vi "Dashboard Main.vi"() -> ()   [LabVIEW 2018]
uses:
  <vilib>/Utility/miscctls.llb/LVRowAndColumnTypeDef.ctl
  <vilib>/event_ctls.llb/eventvkey.ctl
  <vilib>/Rock Robotics/Network Tables/NT Read Numeric Array.vi
  <vilib>/Rock Robotics/WPI/Dashboard/WPI_DashboardLogging Global.vi
panel:
  in  "Camera Settings Right":T1={"Frame Rate"=30, "Compression"=30, "Size"=1, "DB Camera Config"=FALSE} {"Frame Rate" scale=1.0..30.0; "Compression" scale=100.0..-1.0; "Size" items=["640x480", "320x240", "160x120"]}
  in  "Camera Name Right":string(combo)="No Camera Selection"
  out "Camera Perf":string
  in  "Camera Settings":T1={"Frame Rate"=30, "Compression"=30, "Size"=1, "DB Camera Config"=FALSE} {"Frame Rate" scale=1.0..30.0; "Compression" scale=100.0..-1.0; "Size" items=["640x480", "320x240", "160x120"]}
  in  "TCP":refnum<k5>
  in  "Rec Mode":enum32{"Stop", "Record", "Playback"}(radio)
  out "Robot IP":string
  out "Image Message":string="Timeout in Camera Communications"
  in  "Dashboard Tab":T2(tab)
  in  ".Avg Factor":i32=20
  in  "Recognition Limits":T3={"x1 (L) low"=31.0, "x1 (L) high"=71.0, "y1 (L) low "=131.0, "y1 (L) high"=171.0, "x2 (L) low"=249.0, "x2 (L) high"=289.0, "y2 (L) low"=133.0, "y2 (L) high"=173.0}
  out "y1 (L)":dbl
  out "x1 (L)":dbl
  in  "Enable Vision\nProcessing":bool
  out "y2 (R)":dbl
  out "x2 (L)":dbl
  in  "Photo\nStore Rate":u32=100
  in  "Reset":bool
  in  "# New Images\nto Store":i32=1
  in  "Start\nStoring":bool
  out "Total Stored\nSince Reset":i32
  in  "Select Auto":string(combo)="Select Autonomous ..."
  out "NT Connection":bool
  out "MotorChart R":cluster{"Numeric":dbl, "Numeric":dbl}(graph)
  out "MotorChart L":cluster{"Numeric":dbl, "Numeric":dbl}(graph)
  out "MotorSliders R":cluster{"MotorSlide1":dbl, "MotorSlide2":dbl} {"MotorSlide2" scale=-1.0..1.0 scale format="%#_2e"; "MotorSlide1" scale=-1.0..1.0 scale format="%#_2e"}
  out "MotorSliders L":cluster{"MotorSlide1":dbl, "MotorSlide2":dbl} {"MotorSlide2" scale=-1.0..1.0 scale format="%#_2e"; "MotorSlide1" scale=-1.0..1.0 scale format="%#_2e"}
  out "Gyro":dbl(knob) scale=0.0..360.0
  out "JS1 Z":dbl(slide) scale=-1.0..1.0 scale format="%#_2e"
  out "JS1 Graph":cluster{"X":dbl, "Y":dbl}[](graph)
  out "JS1 Buttons":T4
  out "JS2 Z":dbl(slide) scale=-1.0..1.0 scale format="%#_2e"
  out "JS2 Graph":cluster{"X":dbl, "Y":dbl}[](graph)
  out "JS2 Buttons":T4
  out "Mode":T5(ring)=enum."Auto Disabled"
  out "Right Camera Perf":cluster{"Bandwidth (Mbps)":dbl, "FPS":dbl}
  out "Camera Image Right":T6(plugin-control)
  in  "DB/String 9":string
  in  "DB/String 8":string
  in  "DB/String 7":string
  in  "DB/String 6":string
  in  "DB/String 5":string
  in  "DB/String 4":string
  in  "DB/String 3":string
  in  "DB/String 2":string
  in  "DB/String 1":string
  in  "DB/String 0":string
  in  "DB/Slider 0":dbl(slide) scale=0.0..5.0
  in  "DB/Slider 1":dbl(slide) scale=0.0..5.0
  in  "DB/Slider 2":dbl(slide) scale=0.0..5.0
  in  "DB/Slider 3":dbl(slide) scale=0.0..5.0
  out "DB/LED 3":bool
  out "DB/LED 2":bool
  out "DB/LED 1":bool
  out "DB/LED 0":bool
  in  "DB/Button 3":bool
  in  "DB/Button 2":bool
  in  "DB/Button 1":bool
  in  "DB/Button 0":bool caption="New Name"
  in  "Test Slider":dbl(slide) scale=0.0..100.0 scale format="%#_3g"
  in  "On/Off":bool caption="Solenoid"
  in  "Test Name":u16(ring) items=["Select the test to run..."]
  in  "Test Tree":string(tree)
  in  "Motor":cluster{"Value":dbl, "Enable":bool} {"Value" scale=-1.0..1.0 scale format="%#_3g"}
  out "Progress":T7 {"Test Progress" scale=0.0..100.0}
  in  "Rev/Fwd":cluster{"Forward":bool, "Reverse":bool}
  in  "Test Ring":u16(ring) items=["Monochrome", "Color"]
  out "Cmd Status":string
  in  "Execute Command":bool
  in  "Command Params":string[][](table)
  in  "Command Selection":i32(listbox)
  in  "CheckList":i32(listbox)
  out "Tree":string(tree)
  out "Camera Image":T6(plugin-control)
  out "Background":bool
  in  "Camera Name":string(combo)="No Camera Selection"
  # "HW"
  # "HW"
  # "Joysticks"
  # "Drive Motors"
  # "Front"
  # "Right"
  # "Left"
  # "Back"
  # "This tab is a great place for autonomous settings and robot-specific values.\nPlace controls and indicators inside this tab and match name to\nDashboard Variables on robot. You can also delete this comment."
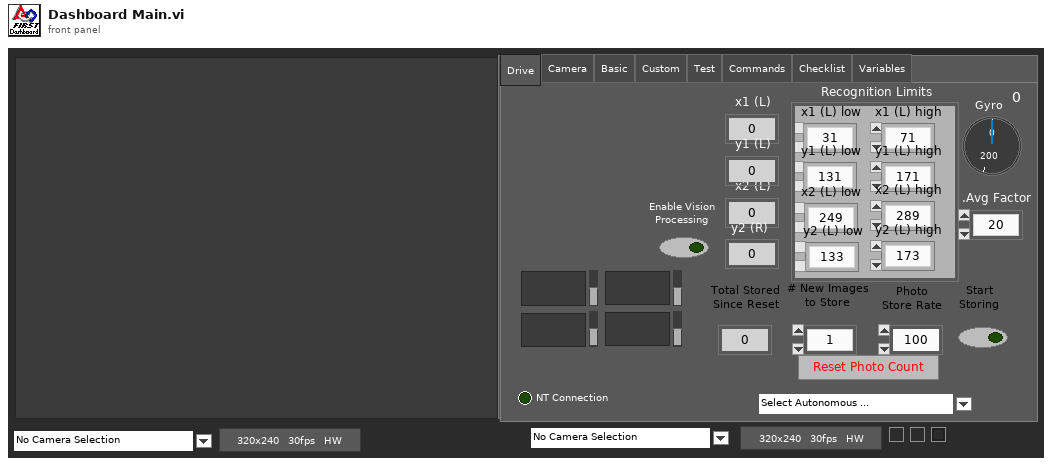
[diagram p1: front panel]
types:
  T1 = cluster{"Frame Rate":i32, "Compression":i32, "Size":u16, "DB Camera Config":bool}
  T2 = enum32{"Drive", "Camera", "Basic", "Custom", "Test", "Commands", "Checklist", "Variables"}
  T3 = cluster{"x1 (L) low":dbl, "x1 (L) high":dbl, "y1 (L) low ":dbl, "y1 (L) high":dbl, "x2 (L) low":dbl, "x2 (L) high":dbl, "y2 (L) low":dbl, "y2 (L) high":dbl}
  T4 = cluster{bool, bool, bool, bool, bool, bool, bool, bool, bool, bool, bool, bool}
  T5 = enum8{"Tele-Op Disabled", "Tele-Op Enabled", "Auto Disabled", "Auto Enabled", "Test Disabled", "Test Enabled", "Disconnected", "No Code", "E-Stop"}
  T6 = typedef "IMAQ Image.ctl" = refnum<image>
  T7 = cluster{"Test Progress":u8, "Test Progress Text":string}
  T8 = cluster{"Save Path":path, "Interval (s)":dbl, "Keep":i32}
  T9 = typedef "Image Type" = u32
  T10 = cluster{"IDs":cluster{"RPC field ID":u16, "Unique ID":u16}, "String":string}
  T11 = cluster{"Error Strings":string, "Disable Counts":cluster{u16, u16}, "Rail Faults":cluster{u16, u16, u16}, "Robot IP":string, "DB Mode":u8, "Event Info":cluster{"Name":string, "Type":u8, "Number":u16, "Replay":u8}}
  T12 = cluster{"Storage":cluster{"Disk Free":u64, "RAM Block":u32, "RAM free":u32}, "CPU Utilization":cluster{"CPU % ISR":sgl, "CPU % Time Crit":sgl, "CPU % Timed Str":sgl, "CPU % High":sgl, "CPU % Above":sgl, "CPU % Normal":sgl, "CPU % Low":sgl}, "CAN":cluster{"% Bus Utilization":sgl, "Bus Off Cnt":u32, "TX_FIFO Full Cnt":u32, "Receive Error Cnt":u8, "Transmit Error Cnt":u8}, "HID":cluster{"HID Outputs":u32, "Rumble Low":u16, "Rumble High":u16}[]}
  T13 = cluster{"Status bits":cluster{"Test Mode":bool, "Autonomous":bool, "Enabled":bool, "Code Start":bool, "Brownout":bool, "Reserved 2":bool, "Reserved 3":bool, "E-Stop":bool}, "Code Trace":cluster{"Disabled":bool, "TeleOp":bool, "Auto":bool, "Test":bool}, "Controller Type":enum16{"unknown", "cRIO", "roboRio"}, "Code?":enum16{"unknown", "noCode", "code"}, "Battery V":dbl}
  T14 = cluster{"Control Bits":cluster{"TestMode":bool, "Autonomous":bool, "Enabled":bool, "FMS Present":bool, bool, bool, bool, "E-Stop":bool}, "Team Station ":u8, "Countdown":sgl, "Joystick Values":cluster{"Axes":dbl[], "Buttons":bool[], "POVs":i16[]}[]}
  T15 = cluster{"Axes":dbl[], "Buttons":bool[], "POVs":i16[]}[]
  T16 = cluster{"Axes":dbl[], "Buttons":bool[], "POVs":i16[]}
  T17 = cluster{"Buttons[0]":bool, "Buttons[1]":bool, "Buttons[2]":bool, "Buttons[3]":bool, "Buttons[4]":bool, "Buttons[5]":bool, "Buttons[6]":bool, "Buttons[7]":bool, "Buttons[8]":bool, "Buttons[9]":bool, "Buttons[10]":bool, "Buttons[11]":bool}
  T18 = cluster{"Camera Image":refnum<vi>, "Dashboard Tab":refnum<vi>, "Background":refnum<vi>, "Rec Mode":refnum<vi>, "Test Slider":refnum<vi>, "On/Off ":refnum<vi>, "Test Ring":refnum<vi>, "Rev/Fwd":refnum<vi>, "Test Name":refnum<vi>, "Motor":refnum<vi>, "Progress":refnum<vi>, "CheckList":refnum<vi>, "Tree":refnum<vi>, "Test Tree":refnum<vi>, "Command Params":refnum<vi>, "Command Selection":refnum<vi>, "Execute Command":refnum<vi>, "Cmd Status":refnum<vi>, "Camera Settings":refnum<vi>, "Camera Name":refnum<vi>, "Camera Perf":refnum<vi>, "Camera Settings Right":refnum<vi>, "Camera Name Right":refnum<vi>, "Camera Image Right":refnum<vi>}
  T19 = cluster{"Global Rectangle":i32[], "Contours":cluster{"Contour Type":u32, "ROI Type":u32, "Points":i32[]}[]}
  T20 = cluster{"Camera Name":string, string, "Saved DB Images Info":cluster{"Save Path":path, "Interval (s)":dbl, "Keep":i32}}
  T21 = cluster{"Position":cluster{"x":sgl, "y":sgl}, "Angle":sgl, "Scale":sgl, "Score":sgl, "Bounding Box":cluster{"x":sgl, "y":sgl}[]}[]
  T22 = typedef "IMAQ GM Match Report.ctl" = cluster{"Position":cluster{"x":sgl, "y":sgl}, "Angle":sgl, "Scale":sgl, "Score":sgl, "Bounding Box":cluster{"x":sgl, "y":sgl}[], "Contrast Reversed":bool, "Occlusion %":sgl, "Template Target Curve Score":sgl, "Target Template Curve Score":sgl, "Correlation Score":sgl}
  T23 = cluster{"Position":cluster{"x":sgl, "y":sgl}, "Angle":sgl, "Scale":sgl, "Score":sgl, "Bounding Box":cluster{"x":sgl, "y":sgl}[]}
  T24 = cluster{"Camera Name Right":string, string, "Saved DB Images Info":cluster{"Save Path":path, "Interval (s)":dbl, "Keep":i32}}
  T25 = cluster{"Operation":enum16{"Update", "Clear"}, "Color Box":u32}[]
  T26 = typedef "eventvkey.ctl" = enum16{"ASCII", "Enter", "Return", "Shift", "Ctrl", "Alt", "Cmd", "Opt", "Caps", "NumLock", "Clear", "Break", "Up", "Down", "Left", "Right", "Insert", "Delete", "Home", "End", "PageUp", "PageDown", "Escape", "Help", "Pause", "ScrollLock", "F1", "F2", "F3", "F4", "F5", "F6", "F7", "F8", "F9", "F10", "F11", "F12", "F13", "F14", "F15", "F16", "F17", "F18", "F19", "F20", "F21", "F22", "F23", "F24", "Play", "VolumeUp", "VolumeDown", "Mute", "Two Byte Char"}
  T27 = cluster{"Image Size":bool, "Image Type":bool, "Pixel Value":bool, "ROI Information":bool, "Zoom Factor":bool}
  T28 = cluster{"Operation":enum16{"Update", "Clear"}, "Color Box":u32}
  T29 = typedef "LVRowAndColumnTypeDef.ctl" = cluster{"Row":i32, "Column":i32}
  T30 = cluster{"Shift":bool, "Ctrl":bool, "Alt":bool, "Cmd":bool, "Opt":bool}
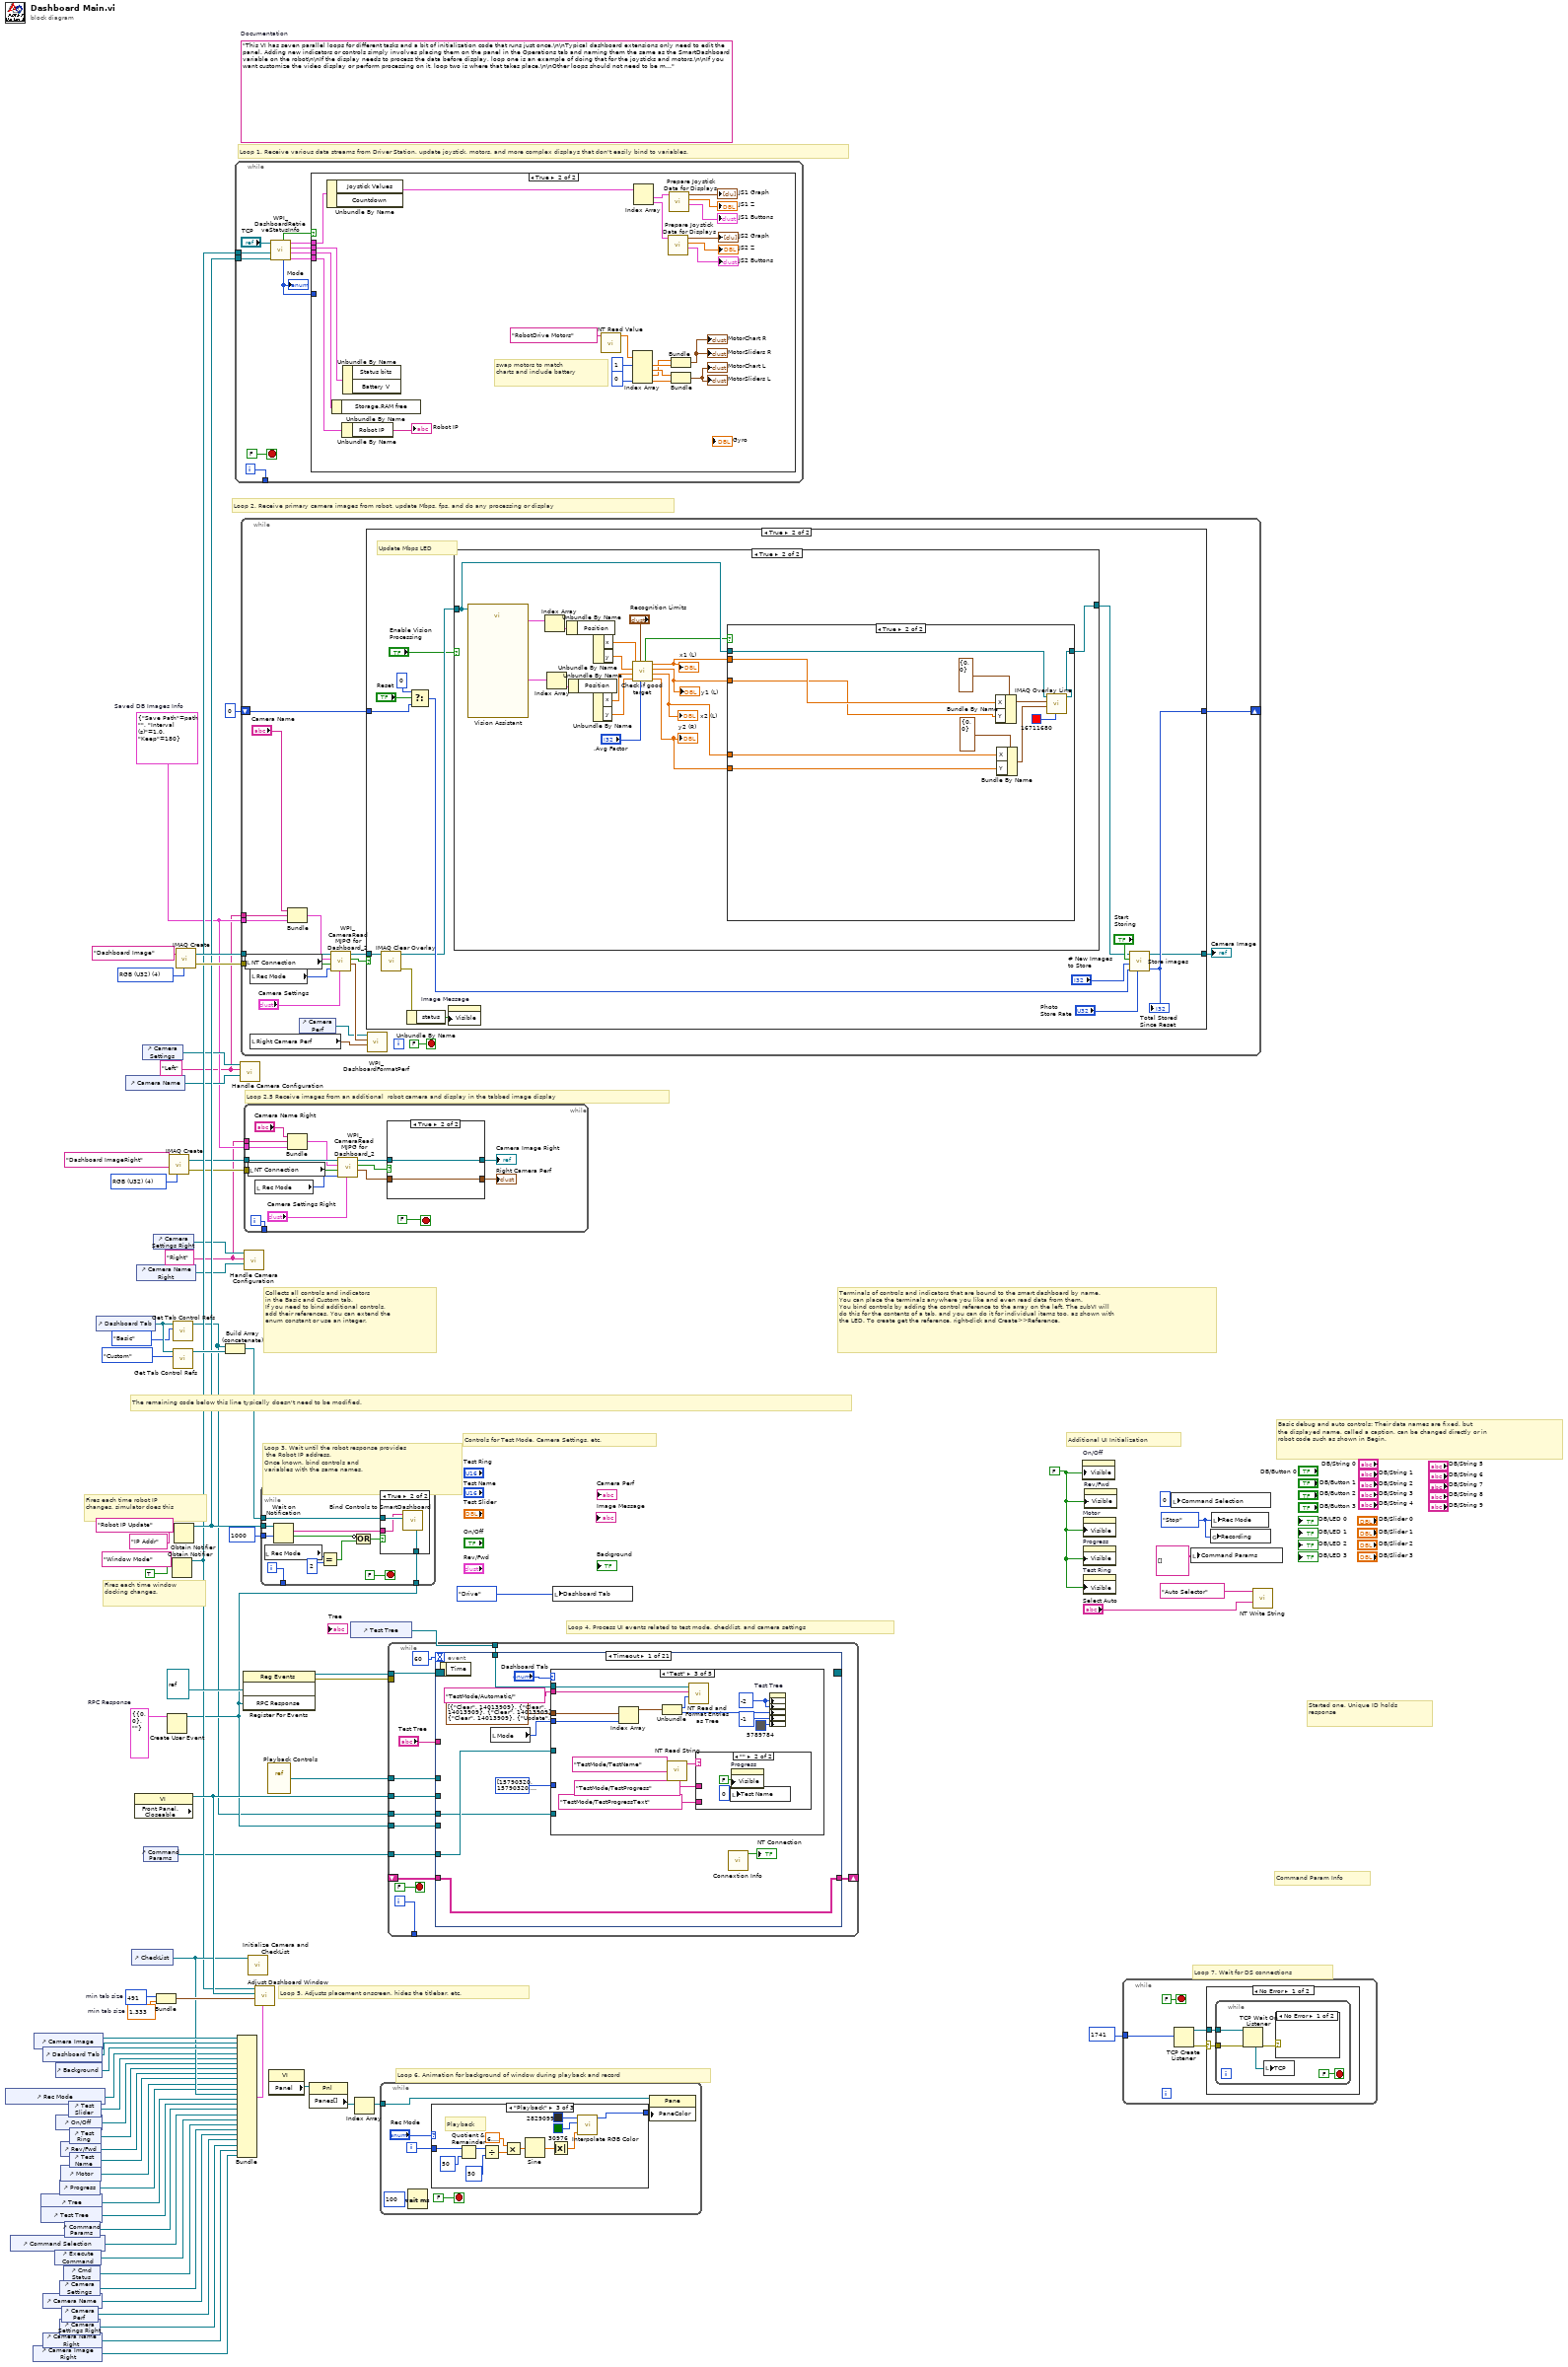
[diagram p0: block diagram]
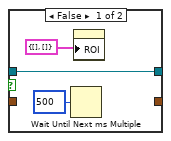
[diagram p2: hidden frame]
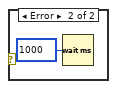
[diagram p3: hidden frame]
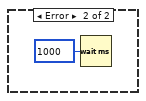
[diagram p4: hidden frame]
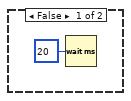
[diagram p5: hidden frame]
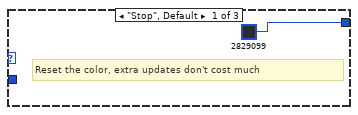
[diagram p6: hidden frame]
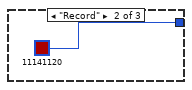
[diagram p7: hidden frame]
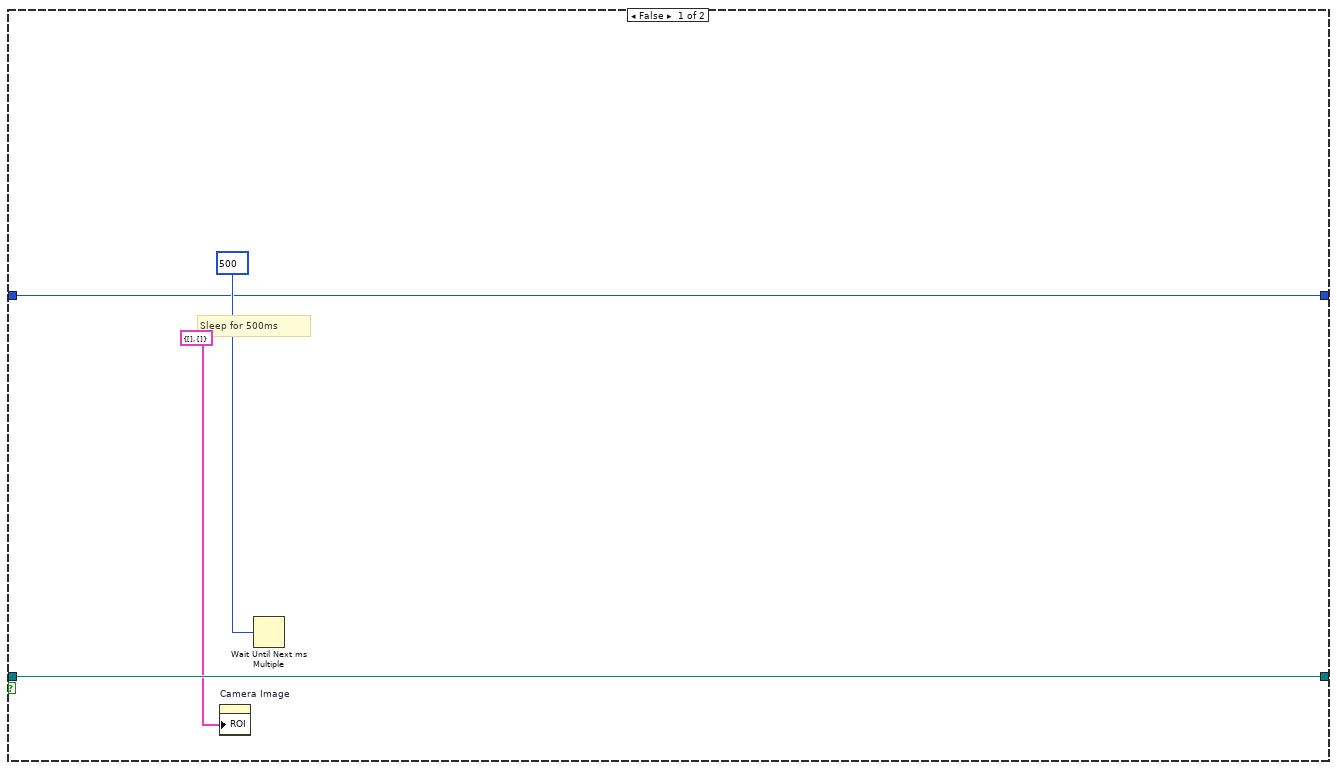
[diagram p9: hidden frame]
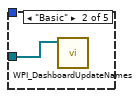
[diagram p13: hidden frame]
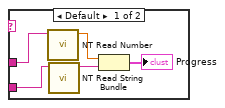
[diagram p14: hidden frame]
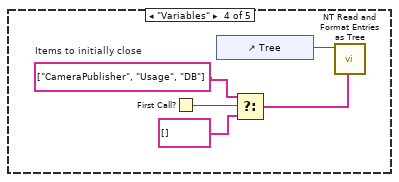
[diagram p15: hidden frame]
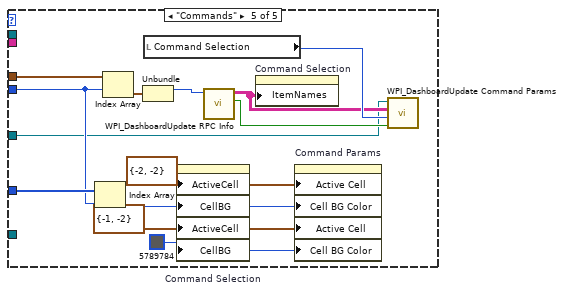
[diagram p16: hidden frame]
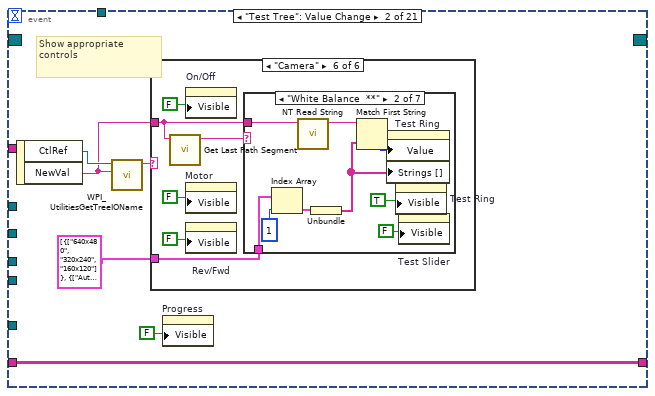
[diagram p17: hidden frame]
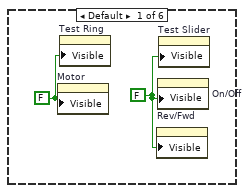
[diagram p18: hidden frame]
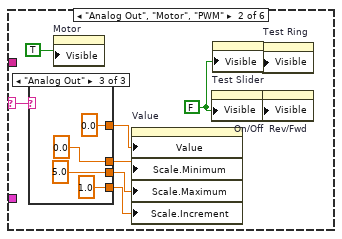
[diagram p19: hidden frame]
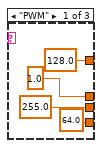
[diagram p20: hidden frame]
diagram:
  w4 = T8 {"Save Path"=path "", "Interval (s)"=1.0, "Keep"=180}  # Saved DB Images Info
  w3 = "Right"
  w2 = "Left"
  w14 = T9 4 items=["Grayscale (U8)", "Grayscale (I16)", "Grayscale (SGL)", "Complex (CSG)", "RGB (U32)", "HSL (U32)", "RGB (U64)"] ("Image Type")
  w30 = T10 {"IDs"={"RPC field ID"=0, "Unique ID"=0}, "String"=""}  # RPC Response
  w53 = 491  # min tab size
  w52 = 1.333  # min tab size
  w60 = enum32{"Stop", "Record", "Playback"}."Stop" ("Rec Mode")
  w37 = FALSE ("Visible")
  (unwired) "This VI has seven parallel loops for different tasks and a bit of initialization code that runs just once.\n\nTypical dashboard extensions only need to edit the panel. Adding new indicators or controls simply involves placing them on the panel in the Operations tab and naming them the same as the SmartDashboard variable on the robot\n\nIf the display needs to process the data before display, loop one is an example of doing that for the joysticks and motors.\n\nIf you want customize the video display or perform processing on it, loop two is where that takes place.\n\nOther loops should not need to be modified. They are pretty standard, and document the task they perform."  # Documentation
  w77 = T9 4 items=["Grayscale (U8)", "Grayscale (I16)", "Grayscale (SGL)", "Complex (CSG)", "RGB (U32)", "HSL (U32)", "RGB (U64)"] ("Image Type")
  # "Loop 2.5 Receive images from an additional  robot camera and display in the tabbed image display"
  # "Command Param Info"
  # "Started one, Unique ID holds\nresponse"
  # "Loop 7. Wait for DS connections"
  # "Basic debug and auto controls: Their data names are fixed, but\nthe displayed name, called a caption, can be changed directly or in\nrobot code such as shown in Begin."
  # "Controls for Test Mode, Camera Settings, etc."
  # "Additional UI Initialization"
  # "Loop 6. Animation for background of window during playback and record"
  # "Fires each time robot IP\nchanges, simulator does this"
  # "Fires each time window\ndocking changes."
  # "Collects all controls and indicators\nin the Basic and Custom tab.\nIf you need to bind additional controls,\nadd their references. You can extend the\nenum constant or use an integer."
  # "The remaining code below this line typically doesn't need to be modified."
  # "Loop 4. Process UI events related to test mode, checklist, and camera settings"
  # "Terminals of controls and indicators that are bound to the smart dashboard by name.\nYou can place the terminals anywhere you like and even read data from them.\nYou bind controls by adding the control reference to the array on the left. The subVI will\ndo this for the contents of a tab, and you can do it for individual items too, as shown with\nthe LED. To create get the reference, right-click and Create>>Reference."
  # "Loop 3. Wait until the robot response provides\n the Robot IP address.\nOnce known, bind controls and\nvariables with the same names."
  # "Loop 5. Adjusts placement onscreen, hides the titlebar, etc."
  # "Loop 1. Receive various data streams from Driver Station, update joystick, motors, and more complex displays that don't easily bind to variables."
  # "Loop 2. Receive primary camera images from robot, update Mbps, fps, and do any processing or display"
  n1 = control-ref of="Rec Mode"() -> (w43:refnum<vi>)
  n2 = control-ref of="Command Selection"() -> (w29:refnum<vi>)
  n3 = control-ref of="Camera Image Right"() -> (w7:refnum<vi>)
  n4 = control-ref of="Camera Image"() -> (w55:refnum<vi>)
  n5 = control-ref of="Tree"() -> (w47:refnum<vi>)
  n6 = control-ref of="Test Tree"() -> (w46:refnum<vi>)
  n7 = control-ref of="Camera Name"() -> (w20:refnum<vi>)
  n8 = control-ref of="Camera Name Right"() -> (w8:refnum<vi>)
  n9 = control-ref of="Dashboard Tab"() -> (w54:refnum<vi>)
  n10 = control-ref of="Execute Command"() -> (w31:refnum<vi>)
  n11 = control-ref of="Background"() -> (w50:refnum<vi>)
  n12 = control-ref of="On/Off"() -> (w41:refnum<vi>)
  n13 = control-ref of="Progress"() -> (w38:refnum<vi>)
  n14 = control-ref of="Camera Settings"() -> (w21:refnum<vi>)
  n15 = control-ref of="Camera Settings Right"() -> (w9:refnum<vi>)
  n16 = control-ref of="Rev/Fwd"() -> (w39:refnum<vi>)
  n17 = control-ref of="Motor"() -> (w44:refnum<vi>)
  n18 = control-ref of="Camera Perf"() -> (w19:refnum<vi>)
  n19 = control-ref of="Cmd Status"() -> (w25:refnum<vi>)
  n20 = control-ref of="Command Params"() -> (w32:refnum<vi>)
  n21 = control-ref of="Test Slider"() -> (w42:refnum<vi>)
  n22 = control-ref of="Test Ring"() -> (w40:refnum<vi>)
  n23 = control-ref of="Test Name"() -> (w45:refnum<vi>)
  n24 = control-ref of="Dashboard Tab"() -> (w58:refnum<vi>)
  n25 = control-ref of="Camera Name"() -> (w22:refnum<vi>)
  n26 = control-ref of="CheckList"() -> (w48:refnum<vi>)
  n27 = property class="VI" props=["Front Panel.Closeable"]() -> (reference out=w59:refnum<vi>)  [unwired: 2 in, 2 out]
  n28 = control-ref of="Camera Name Right"() -> (w10:refnum<vi>)
  n29 = control-ref of="Camera Settings"() -> (w23:refnum<vi>)
  n30 = control-ref of="Command Params"() -> (w24:refnum<vi>)
  n31 = control-ref of="Camera Settings Right"() -> (w11:refnum<vi>)
  n32 = Bundle("min tab size"=w53, "min tab size"=w52) -> (w51:cluster{"min tab size":i32, "min tab size":dbl})  [unwired: 1 in]
  n33 = Create User Event(user event datatype=w30) -> (user event=w26:refnum<user-event>)  [unwired: 1 in, 1 out]
  n34 = call "IMAQ Create"("Image Name"="Dashboard ImageRight", "Image Type"=w14) -> ("New Image"=w13:T6, "error out"=w12:errorcluster)  [unwired: 2 in, 1 out]
  n35 = Obtain Notifier(name (unnamed)="Window Mode", notification data type=TRUE) -> (notifier out=w35:refnum<notifier>)  [unwired: 2 in, 2 out]
  n36 = call <vilib>:"Get Tab Control Refs.vi"("Page Index"=T2."Basic" ("Dashboard Tab"), "TabControl in"=w58) -> ("ControlsOnPage"=w18:refnum<vi>[])  [unwired: 9 in]
  n37 = call <vilib>:"Get Tab Control Refs.vi"("Page Index"=T2."Custom" ("Dashboard Tab"), "TabControl in"=w58) -> ("ControlsOnPage"=w57:refnum<vi>[])  [unwired: 9 in]
  n38 = Obtain Notifier(name (unnamed)="Robot IP Update", notification data type="IP Addr" ("name (unnamed)")) -> (notifier out=w36:refnum<notifier>)  [unwired: 2 in, 2 out]
  n39 = call "IMAQ Create"("Image Name"="Dashboard Image", "Image Type"=w77) -> ("New Image"=w75:T6, "error out"=w74:errorcluster)  [unwired: 2 in, 1 out]
  n40 = Build Array (concatenate)(w18, w57) -> (w56:refnum<vi>[])
  n41 = while {
    tunnel: [w87] -> _
    tunnel: w36 -> [w81]
    tunnel: w35 -> [w78]
    i -> [w87]
    stop <- FALSE stop-if-true
    n42 = call <vilib>:"WPI_DashboardRetrieveStatusInfo.vi"("Binding Refnum"=w81, "Window Mode Notifier"=w78, "TCP Cnx"="TCP") -> ("Power and Errors"=w82:T11, "Robot Metrics"=w85:T12, "Status Info"=w86:T13, "Control Info"=w83:T14, "Robot Mode"=w80:T5, "Process?"=w84:bool)  [unwired: 3 in]
    "Mode" <- w80
    n43 = case shown="True" w84 {
      tunnel: w86 -> [_ w113]
      tunnel: w85 -> [_ w112]
      tunnel: w83 -> [_ w111]
      tunnel: w82 -> [_ w110]
      tunnel: w80 -> [_ _]
      frame False {
        n44 = Wait (ms)(milliseconds to wait=u32 20) -> ()  [unwired: 1 out]
      }
      frame True {
        # "swap motors to match\ncharts and include battery"
        n45 = Unbundle By Name(w111) -> ("Joystick Values"=w101:T15)  [unwired: 1 out]
        n46 = Unbundle By Name(w112) -> ()  [unwired: 1 out]
        n47 = Unbundle By Name(w110) -> ("Robot IP"=→"Robot IP":string)
        n48 = Unbundle By Name(w113) -> ()  [unwired: 2 out]
        n49 = call-poly <vilib>:"NT Read Value.vi"("Name"="RobotDrive Motors") -> ("Numeric Array"=w91:dbl[])  [unwired: 9 in, 1 out]
        n50 = Index Array(array=w91, index #1=1, index #4=0) -> (element #1=w105:dbl, element #2=w106:dbl, element #3=w104:dbl, element #4=w109:dbl)  [unwired: 2 in]
        n51 = Index Array(array=w101) -> (element #1=w100:T16, element #2=w96:T16)  [unwired: 2 in]
        n52 = call "Prepare Joystick Data for Displays.vi"("Joystick Values"=w96) -> ("Buttons"=→"JS2 Buttons":T17, "Z Axis"=→"JS2 Z":dbl, "Cartesian Data"=→"JS2 Graph":cluster{"X axis":dbl, "X axis":dbl}[])  [unwired: 8 in]
        n53 = call "Prepare Joystick Data for Displays.vi"("Joystick Values"=w100) -> ("Buttons"=→"JS1 Buttons":T17, "Z Axis"=→"JS1 Z":dbl, "Cartesian Data"=→"JS1 Graph":cluster{"X axis":dbl, "X axis":dbl}[])  [unwired: 8 in]
        n54 = Bundle("Numeric"=w104, "Numeric"=w105) -> (→"MotorChart R" →"MotorSliders R":cluster{"Numeric":dbl, "Numeric":dbl})  [unwired: 1 in]
        n55 = Bundle("Numeric"=w106, "Numeric"=w109) -> (→"MotorChart L" →"MotorSliders L":cluster{"Numeric":dbl, "Numeric":dbl})  [unwired: 1 in]
      }
    }
  }
  n56 = Bundle("Camera Image"=w55, "Dashboard Tab"=w54, "Background"=w50, "Rec Mode"=w43, "Test Slider"=w42, "On/Off"=w41, "Test Ring"=w40, "Rev/Fwd"=w39, "Test Name"=w45, "Motor"=w44, "Progress"=w38, "CheckList"=w48, "Tree"=w47, "Test Tree"=w46, "Command Params"=w32, "Command Selection"=w29, "Execute Command"=w31, "Cmd Status"=w25, "Camera Settings"=w21, "Camera Name"=w20, "Camera Perf"=w19, "Camera Settings Right"=w9, "Camera Name Right"=w8, "Camera Image Right"=w7) -> (w49:T18)  [unwired: 1 in]
  n57 = call "Handle Camera Configuration.vi"("CameraNameRef"=w22, "Display Name"=w2, "ClusterRef"=w23) -> ()  [unwired: 9 in]
  n58 = while {
    tunnel: w75 -> [w129]
    tunnel: w74 -> [_]
    tunnel: w4 -> [w122]
    tunnel: w2 -> [w119]
    shift-right: [w115] -> _
    shift-left: 0 -> [w114]
    stop <- FALSE stop-if-true
    n59 = local read "NT Connection"() -> (w123:bool)
    n60 = local read "Right Camera Perf"() -> (w117:cluster{"Bandwidth (Mbps)":dbl, "FPS":dbl})
    n61 = local read "Rec Mode"() -> (w126:enum32{"Stop", "Record", "Playback"})
    n62 = Bundle("Camera Name"="Camera Name", w119, "Saved DB Images Info"=w122) -> (w121:T20)  [unwired: 1 in]
    n63 = control-ref of="Camera Perf"() -> (w116:refnum<vi>)
    n64 = call <vilib>:"WPI_CameraRead MJPG for Dashboard_2.vi"("Camera Settings"="Camera Settings", "Rec Mode"=w126, "NT Connection"=w123, "Capture Info"=w121, "Image in"=w129) -> ("perf info"=w118:cluster{"Bandwidth (Mbps)":dbl, "fps":dbl}, "Active"=w127:bool, "Image\\ out"=w128:T6)  [unwired: 4 in]
    n65 = case shown="True" w127 {
      tunnel: w128 -> [w133 w147]
      tunnel: [w133 w136] -> w124
      tunnel: [w131 w146] -> w115
      tunnel: w114 -> [w131 w143]
      frame False {
        # "Sleep for 500ms"
        n66 = property on="Camera Image" class="ImageControl"("ROI"=T19 {"Global Rectangle"=[], "Contours"=[]}) -> ()  [unwired: 2 in, 2 out]
        n67 = Wait Until Next ms Multiple(millisecond multiple=u32 500) -> ()  [unwired: 1 out]
      }
      frame True {
        # "Update Mbps LED"
        n68 = call "IMAQ Clear Overlay"("Image"=w147) -> ("error out"=w148:errorcluster, "Image Out"=w141:T6)  [unwired: 2 in, 7 out]
        n69 = Unbundle By Name(w148) -> ("status"=w149:bool)
        n70 = Select(t=0, s="Reset", f=w143) -> (s? t:f=w142:i32)
        n71 = property on="Image Message" class="Str"("Visible"=w149) -> ()  [unwired: 2 in, 2 out]
        n72 = case shown="True" "Enable Vision\nProcessing" {
          tunnel: w141 -> [w150 w167]
          tunnel: [w150 w169] -> w137
          frame False {
          }
          frame True {
            n73 = call "Vision Assistant"("Image In"=w167) -> ("Calibrated Matches (Pattern Matching 2)"=w168:T21, "Calibrated Matches (Pattern Matching 1)"=w166:T22[])  [unwired: 23 in, 2 out]
            n74 = Index Array(array=w166) -> (element=w165:T22)  [unwired: 1 in]
            n75 = Index Array(array=w168) -> (element=w162:T23)  [unwired: 1 in]
            n76 = Unbundle By Name(w165) -> ("Position"=w164:cluster{"x":sgl, "y":sgl})
            n77 = Unbundle By Name(w162) -> ("Position"=w163:cluster{"x":sgl, "y":sgl})
            n78 = Unbundle By Name(w163) -> ("x"=w159:sgl, "y"=w158:sgl)
            n79 = Unbundle By Name(w164) -> ("x"=w161:sgl, "y"=w160:sgl)
            n80 = call "Check if good target.vi"("Avg Factor"=".Avg Factor", "Limits"="Recognition Limits", "y2-R"=w158, "x2-R"=w159, "y1-L"=w160, "x1-L"=w161) -> ("y2 (R) out"=w151:dbl, "x2 (L) out"=w152:dbl, "y1 (L) out"=w153:dbl, "x1 (L) out"=w154:dbl, "Good target?"=w157:bool)  [unwired: 1 in]
            "x2 (L)" <- w152
            "y2 (R)" <- w151
            "x1 (L)" <- w154
            "y1 (L)" <- w153
            n81 = case shown="True" w157 {
              tunnel: w167 -> [w170 w181]
              tunnel: [w170 w172] -> w169
              tunnel: w154 -> [_ w176]
              tunnel: w153 -> [_ w175]
              tunnel: w152 -> [_ w174]
              tunnel: w151 -> [_ w173]
              frame False {
              }
              frame True {
                n82 = Bundle By Name(cluster=cluster{"X":i32, "Y":i32} {"X"=0, "Y"=0} ("Start Point"), "X"=w176, "Y"=w175) -> (w180:cluster{"X":i32, "Y":i32})
                n83 = Bundle By Name(cluster=cluster{"X":i32, "Y":i32} {"X"=0, "Y"=0} ("Start Point"), "X"=w174, "Y"=w173) -> (w178:cluster{"X":i32, "Y":i32})
                n84 = call "IMAQ Overlay Line"("Color"=u32 16711680, "End Point"=w178, "Start Point"=w180, "Image"=w181) -> ("Image Out"=w172:T6)  [unwired: 6 in, 1 out]
              }
            }
          }
        }
        n85 = call "Store images.vi"("ms Capture Rate"="Photo\nStore Rate", "# Total images IN"=w142, "# new images to capture"="# New Images\nto Store", "Store # Images?"="Start\nStoring", "Image"=w137) -> ("Total images OUT"=w146:i32, "Image Out"=w136:T6)  [unwired: 5 in]
        "Total Stored\nSince Reset" <- w146
      }
    }
    "Camera Image" <- w124
    n86 = call <vilib>:"WPI_DashboardFormatPerf.vi"("Right Camera Perf"=w117, "Performance"=w118, "String in"=w116) -> ()  [unwired: 9 in]
  }
  n87 = register-events(refnum<vi> refnum, w26) -> (reference out=w64:refnum<event-registration>, error out=w63:errorcluster)  [unwired: 2 in]
  n88 = while {
    tunnel: w13 -> [w196]
    tunnel: w12 -> [_]
    tunnel: [w191] -> _
    tunnel: w4 -> [w187]
    tunnel: w3 -> [w184]
    i -> [w191]
    stop <- FALSE stop-if-true
    n89 = local read "NT Connection"() -> (w188:bool)
    n90 = local read "Rec Mode"() -> (w195:enum32{"Stop", "Record", "Playback"})
    n91 = Bundle("Camera Name Right"="Camera Name Right", w184, "Saved DB Images Info"=w187) -> (w186:T24)  [unwired: 1 in]
    n92 = call <vilib>:"WPI_CameraRead MJPG for Dashboard_2.vi"("Camera Settings"="Camera Settings Right", "Rec Mode"=w195, "NT Connection"=w188, "Capture Info"=w186, "Image in"=w196) -> ("perf info"=w182:cluster{"Bandwidth (Mbps)":dbl, "fps":dbl}, "Active"=w190:bool, "Image\\ out"=w193:T6)  [unwired: 4 in]
    n93 = case shown="True" w190 {
      tunnel: w193 -> [w198 w201]
      tunnel: [w198 w201] -> w189
      tunnel: [_ w200] -> w183
      tunnel: w182 -> [_ w200]
      frame False {
        n94 = Wait Until Next ms Multiple(millisecond multiple=u32 500) -> ()  [unwired: 1 out]
        n95 = property on="Camera Image Right" class="ImageControl"("ROI"=T19 {"Global Rectangle"=[], "Contours"=[]}) -> ()  [unwired: 2 in, 2 out]
      }
      frame True {
      }
    }
    "Camera Image Right" <- w189
    "Right Camera Perf" <- w183
  }
  n96 = call "Handle Camera Configuration.vi"("CameraNameRef"=w10, "Display Name"=w3, "ClusterRef"=w11) -> ()  [unwired: 9 in]
  n97 = call "Initialize Camera and CheckList.vi"("ListBox in"=w48) -> ()  [unwired: 11 in]
  n98 = call "Adjust Dashboard Window.vi"("Sizing Refnums"=w49, "Size Constraints"=w51, "VI"=w59, "WIn Mode"=w35) -> ()  [unwired: 8 in]
  n99 = while {
    tunnel: w56 -> [w213]
    tunnel: w36 -> [w211]
    tunnel: [w209] -> _
    tunnel: u32 1000 ("milliseconds to wait") -> [w208]
    tunnel: w26 -> [w202]
    i -> [w209]
    stop <- FALSE stop-if-true
    n100 = local read "Rec Mode"() -> (w204:enum32{"Stop", "Record", "Playback"})
    n101 = Wait on Notification(notifier=w211, timeout in ms (-1)=w208) -> (notification=w210:string, timed out?=w206:bool)  [unwired: 2 in, 2 out]
    n102 = Equal?(x=w204, y=u16 2 ("Rec Mode")) -> (x = y?=w205:bool)
    n103 = Compound Arithmetic op=OR(invert w206, w205) -> (w207:bool)
    n104 = case shown="True" w207 {
      tunnel: w213 -> [_ w216]
      tunnel: w210 -> [_ w215]
      tunnel: w202 -> [_ w214]
      frame False {
      }
      frame True {
        n105 = call <vilib>:"Bind Controls to SmartDashboard.vi"("RPC ref"=w214, "Bound Control Refs"=w216, "Server IP Address"=w215) -> ()  [unwired: 9 in]
      }
    }
  }
  n106 = vi-ref "Playback Controls.vi"() -> (w65:refnum<vi>)
  n107 = property class="VI"() -> ("Panel"=w67:refnum<vi>)  [unwired: 2 in, 2 out]
  n108 = property class="Pnl"(reference=w67) -> ("Panes[]"=w68:refnum<vi>[])  [unwired: 1 in, 2 out]
  n109 = control-ref of="Test Tree"() -> (w69:refnum<vi>)
  n110 = Index Array(array=w68) -> (element=w66:refnum<vi>)  [unwired: 1 in]
  n111 = while {
    tunnel: w66 -> [w218]
    i -> [w221]
    stop <- FALSE stop-if-true
    n112 = Wait (ms)(milliseconds to wait=u32 100) -> ()  [unwired: 1 out]
    n113 = case shown="\"Playback\"" "Rec Mode" {
      tunnel: w221 -> [_ _ w236]
      tunnel: [u32 2829099 ("Base Color") u32 11141120 ("Target Color") w225] -> w217
      frame "Stop", Default {
        # "Reset the color, extra updates don't cost much"
      }
      frame "Record" {
      }
      frame "Playback" {
        # "Playback"
        n114 = Quotient & Remainder(x=w236, y=u32 50 ("milliseconds to wait")) -> (x-y*floor(x/y)=w232:u32)  [unwired: 1 out]
        n115 = Divide(x=w232, y=u32 50 ("milliseconds to wait")) -> (x/y=w229:dbl)
        n116 = Multiply(x=6.283185307179586, y=w229) -> (x*y=w234:dbl)
        n117 = Sine(x=w234) -> (sin(x)=w233:dbl)
        n118 = Absolute Value(x=w233) -> (abs(x)=w226:dbl)
        n119 = call "Interpolate RGB Color.vi"("Proportion"=w226, "Target Color"=u32 30976, "Base Color"=u32 2829099) -> ("Result Color"=w225:u32)  [unwired: 8 in]
      }
    }
    n120 = property class="Pane"(reference=w218, "PaneColor"=w217) -> ()  [unwired: 1 in, 2 out]
  }
  n121 = while {
    tunnel: [w246] -> _
    tunnel: w69 -> [w245]
    tunnel: w65 -> [w244]
    tunnel: w64 -> [w243]
    tunnel: w63 -> [_]
    tunnel: w59 -> [w242]
    tunnel: w26 -> [w241]
    tunnel: w24 -> [w240]
    shift-right: [w239] -> _
    shift-left: _ -> [w238]
    tunnel: w18 -> [w237]
    i -> [w246]
    stop <- FALSE stop-if-true
    n122 = event shown="[0] Timeout" {
      selector: w243 -> [_ _ _ _ _ _ _ _ _ _ _ _ _ _ _ _ _ _ _ _ _]
      dyn-events: [_ _ _ _ _ _ _ _ _ _ _ _ _ _ _ _ w506 _ _ _ _] -> _
      timeout: u32 60 ("milliseconds to wait") -> [_ _ _ _ _ _ _ _ _ _ _ _ _ _ _ _ _ _ _ _ _]
      tunnel: w245 -> [w258 _ _ _ _ _ _ _ _ _ _ _ _ _ _ _ _ _ _ _ _]
      tunnel: "Test Tree" -> [_ _ _ _ _ _ _ _ _ _ _ w473 w481 w483 w487 w495 _ _ _ _ _]
      tunnel: w244 -> [_ _ _ _ _ _ _ _ _ _ _ _ _ _ _ _ w508 _ w526 _ _]
      tunnel: w242 -> [_ _ _ _ _ _ _ _ _ _ _ _ _ _ _ _ w504 _ _ _ _]
      tunnel: w241 -> [_ _ _ _ _ _ _ _ _ _ _ _ _ _ _ _ w502 _ _ _ _]
      tunnel: w240 -> [w253 _ _ _ _ _ w424 _ _ _ _ _ _ _ _ _ _ _ _ _ _]
      tunnel: [w252 w301 w403 w408 w417 w421 w422 w431 w441 w448 w460 w472 w479 w482 w486 w494 w501 w521 w523 w527 w540] -> w239
      tunnel: w238 -> [w252 w301 w403 w408 w417 w421 w422 _ _ w448 w460 w472 w479 w482 w486 w494 w501 w521 w523 w527 w540]
      tunnel: w237 -> [w250 _ _ _ _ _ _ _ _ _ _ _ _ _ _ _ _ _ _ _ _]
      event Timeout {
        n123 = event-data() -> ()  [unwired: 1 in, 1 out]
        n124 = local read "Mode"() -> (w255:T5)
        n125 = case shown="\"Test\"" "Dashboard Tab" {
          tunnel: w258 -> [_ _ w274 _ _]
          tunnel: "TestMode/Automatic/" ("Name Pattern") -> [_ _ w273 _ _]
          tunnel: T25 [{"Operation"=enum."Clear", "Color Box"=14013909}, {"Operation"=enum."Clear", "Color Box"=14013909}, {"Operation"=enum."Clear", "Color Box"=14013909}, {"Operation"=enum."Clear", "Color Box"=14013909}, {"Operation"=enum."Update", "Color Box"=14013909}, {"Operation"=enum."Update", "Color Box"=16777215}, {"Operation"=enum."Clear", "Color Box"=14013909}, {"Operation"=enum."Clear", "Color Box"=14013909}, {"Operation"=enum."Clear", "Color Box"=14013909}] -> [_ _ w266 _ w294]
          tunnel: w255 -> [_ _ w265 _ w293]
          tunnel: u32[] [15790320, 15790320, 15790320, 15790320, 16777215, 16777215, 15790320, 15790320, 15790320] -> [_ _ _ _ w299]
          tunnel: w253 -> [_ _ _ _ w287]
          tunnel: w250 -> [_ w260 _ _ _]
          frame "Custom", Default {
          }
          frame "Basic" {
            n126 = call <vilib>:"WPI_DashboardUpdateNames.vi"("Controls on Tab"=w260) -> ()  [unwired: 11 in]
          }
          frame "Test" {
            w272 = -2 ("Active Item:Row Number")
            n127 = Index Array(array=w266, index=w265) -> (element=w267:T28)
            n128 = Unbundle(w267) -> ("Operation"=w268:enum16{"Update", "Clear"}, "Color Box"=w269:u32)
            n129 = call <vilib>:"NT Read String.vi"("Name"="TestMode/TestName") -> ("String"=w263:string)  [unwired: 9 in, 1 out]
            n130 = call <vilib>:"NT Read and Format Entries as Tree.vi"("Operation"=w268, "Name Pattern"=w273, "Tree Refnum"=w274) -> ()  [unwired: 7 in, 2 out]
            n131 = case shown="\"\"" w263 {
              tunnel: "TestMode/TestProgress" ("Name") -> [w276 _]
              tunnel: "TestMode/TestProgressText" ("Name") -> [w275 _]
              frame Default {
                n132 = call <vilib>:"NT Read Number.vi"("Name"=w276) -> ("Numeric"=w277:dbl)  [unwired: 9 in, 1 out]
                n133 = call <vilib>:"NT Read String.vi"("Name"=w275) -> ("String"=w278:string)  [unwired: 9 in, 1 out]
                n134 = Bundle("Numeric"=w277, "String"=w278) -> (→"Progress":cluster{"Numeric":dbl, "String":string})  [unwired: 1 in]
              }
              frame "" {
                n135 = local write "Test Name"(u16 0) -> ()
                n136 = property on="Progress" class="Clust (strict)"("Visible"=FALSE) -> ()  [unwired: 2 in, 2 out]
              }
            }
            n137 = property on="Test Tree" class="Tree (strict)"("Active Item Row Number"=w272, "ActiveColNum"=w272, "CellBG"=w269, "Active Item Row Number"=-1 ("Active Item:Row Number"), "CellBG"=u32 5789784 ("Color Box")) -> ()  [unwired: 2 in, 2 out]
          }
          frame "Variables" {
            w284 = string[] ["CameraPublisher", "Usage", "DB"]  # Items to initially close
            n138 = First Call?() -> (First Call?: T/F=w285:bool)
            n139 = control-ref of="Tree"() -> (w286:refnum<vi>)
            n140 = Select(t=w284, s=w285, f=string[] []) -> (s? t:f=w282:string[])
            n141 = call <vilib>:"NT Read and Format Entries as Tree.vi"("Tags to  Close"=w282, "Tree Refnum"=w286) -> ()  [unwired: 8 in, 2 out]
          }
          frame "Commands" {
            w295 = u32 5789784 ("Color Box")
            w296 = T29 {"Row"=-1, "Column"=-2} ("Active Cell:Active Cell")
            w298 = T29 {"Row"=-2, "Column"=-2} ("Active Cell:Active Cell")
            n142 = Index Array(array=w299, index=w293) -> (element=w297:u32)
            n143 = Index Array(array=w294, index=w293) -> (element=w292:T28)
            n144 = Unbundle(w292) -> ("Operation"=w291:enum16{"Update", "Clear"})  [unwired: 1 out]
            n145 = local read "Command Selection"() -> (w290:i32)
            n146 = property on="Command Selection" class="MCListbox (strict)"("ActiveCell"=w298, "CellBG"=w297, "ActiveCell"=w296, "CellBG"=w295) -> ()  [unwired: 2 in, 2 out]
            n147 = call <vilib>:"WPI_DashboardUpdate RPC Info.vi"("Operation"=w291) -> ("update"=w289:bool, "commands"=w288:string[][])  [unwired: 9 in]
            n148 = property on="Command Selection" class="MCListbox (strict)"("ItemNames"=w288) -> ()  [unwired: 2 in, 2 out]
            n149 = property on="Command Params" class="Tbl (strict)"("Active Cell"=w298, "Cell BG Color"=w297, "Active Cell"=w296, "Cell BG Color"=w295) -> ()  [unwired: 2 in, 2 out]
            n150 = call <vilib>:"WPI_DashboardUpdate Command Params.vi"("Update"=w289, "NewVal"=w290, "Commands"=w288, "Param Tbl"=w287) -> ()  [unwired: 7 in, 1 out]
          }
        }
        n151 = call <vilib>:"Connextion Info.vi"() -> ("Connected"=→"NT Connection":bool)  [unwired: 10 in, 1 out]
      }
      event "Test Tree": Value Change {
        # "Show appropriate\ncontrols"
        n152 = event-data() -> ("CtlRef"=w304:refnum<vi>, "NewVal"=w302:string)  [unwired: 1 in]
        n153 = call <vilib>:"WPI_UtilitiesGetTreeIOName.vi"("NewVal"=w302, "TreeControl in"=w304) -> ("I/O Name"=w305:string)  [unwired: 9 in]
        n154 = case shown="\"Camera\"" w305 {
          selector: w305 -> [_ w312 _ w334 w343 _]
          tunnel: w302 -> [_ _ w331 w333 _ w350]
          tunnel: cluster{string[]}[] [{["640x480", "320x240", "160x120"]}, {["Auto", "Fixed indoor", "Fixed outdoor 1", "Fixed outdoor 2", "Fixed fluorescent 1", "Fixed fluorescent 2", "Hold current"]}, {["Auto", "Flicker-free 50 Hz", "Flicker-free 60 Hz", "Hold current"]}, {["None", "Prioritize frame rate", "Prioritize image quality"]}, {["Monochrome", "Color"]}] -> [_ _ _ _ _ w349]
          frame Default {
            w307 = FALSE ("Visible")
            w306 = FALSE ("Visible")
            n155 = property on="Motor" class="Clust (strict)"("Visible"=w306) -> ()  [unwired: 2 in, 2 out]
            n156 = property on="Test Ring" class="Ring (strict)"("Visible"=w306) -> ()  [unwired: 2 in, 2 out]
            n157 = property on="Rev/Fwd" class="Clust (strict)"("Visible"=w307) -> ()  [unwired: 2 in, 2 out]
            n158 = property on="On/Off" class="Bool (strict)"("Visible"=w307) -> ()  [unwired: 2 in, 2 out]
            n159 = property on="Test Slider" class="Slide (strict)"("Visible"=w307) -> ()  [unwired: 2 in, 2 out]
          }
          frame "Analog Out", "Motor", "PWM" {
            w313 = FALSE ("Visible")
            n160 = case shown="\"Analog Out\"" w312 {
              tunnel: [1.0 ("Value") -1.0 ("Value") 0.0 ("Value")] -> w311
              tunnel: [255.0 ("Value") 1.0 ("Value") 5.0 ("Value")] -> w310
              tunnel: [128.0 ("Value") 0.0 ("Value") 0.0 ("Value")] -> w309
              tunnel: [64.0 ("Value") 0.5 ("Value") 1.0 ("Value")] -> w308
              frame "PWM" {
              }
              frame "Motor", Default {
              }
              frame "Analog Out" {
              }
            }
            n161 = property on="Motor" class="Clust (strict)"("Visible"=TRUE) -> ()  [unwired: 2 in, 2 out]
            n162 = property on="Value" class="Slide (strict)"("Value"=w309, "Scale.Minimum"=w311, "Scale.Maximum"=w310, "Scale.Increment"=w308) -> ()  [unwired: 2 in, 2 out]
            n163 = property on="On/Off" class="Bool (strict)"("Visible"=w313) -> ()  [unwired: 2 in, 2 out]
            n164 = property on="Test Slider" class="Slide (strict)"("Visible"=w313) -> ()  [unwired: 2 in, 2 out]
            n165 = property on="Test Ring" class="Ring (strict)"("Visible"=w313) -> ()  [unwired: 2 in, 2 out]
            n166 = property on="Rev/Fwd" class="Clust (strict)"("Visible"=w313) -> ()  [unwired: 2 in, 2 out]
          }
          frame "Servo" {
            w329 = FALSE ("Visible")
            n167 = call <vilib>:"NT Read Number.vi"("Name"=w331) -> ("Numeric"=w330:dbl)  [unwired: 9 in, 1 out]
            n168 = property on="Test Slider" class="Slide (strict)"("Visible"=TRUE, "Scale.Maximum"=170.0 ("Scale.Range:Maximum")) -> ()  [unwired: 2 in, 2 out]
            n169 = local write "Test Slider"(w330) -> ()
            n170 = property on="Motor" class="Clust (strict)"("Visible"=w329) -> ()  [unwired: 2 in, 2 out]
            n171 = property on="Rev/Fwd" class="Clust (strict)"("Visible"=w329) -> ()  [unwired: 2 in, 2 out]
            n172 = property on="On/Off" class="Bool (strict)"("Visible"=w329) -> ()  [unwired: 2 in, 2 out]
            n173 = property on="Test Ring" class="Ring (strict)"("Visible"=w329) -> ()  [unwired: 2 in, 2 out]
          }
          frame "Relay", "Solenoid" {
            w332 = FALSE ("Visible")
            n174 = property on="Motor" class="Clust (strict)"("Visible"=w332) -> ()  [unwired: 2 in, 2 out]
            n175 = property on="Test Slider" class="Slide (strict)"("Visible"=w332) -> ()  [unwired: 2 in, 2 out]
            n176 = Search and Replace String(input string=w333, search string="/Value  **", replace string="/Direction") -> (result string=w339:string)  [unwired: 5 in, 3 out]
            n177 = property on="Test Ring" class="Ring (strict)"("Visible"=w332) -> ()  [unwired: 2 in, 2 out]
            n178 = call <vilib>:"NT Read String.vi"("Name"=w339) -> ("String"=w337:string)  [unwired: 9 in, 1 out]
            n179 = Equal?(x="Both directions", y=w337) -> (x = y?=w335:bool)
            n180 = Not(x=w335) -> (.not. x?=w336:bool)
            n181 = property on="Rev/Fwd" class="Clust (strict)"("Visible"=w335) -> ()  [unwired: 2 in, 2 out]
            n182 = property on="On/Off" class="Bool (strict)"("Visible"=w336, "Caption.Text"=w334) -> ()  [unwired: 2 in, 2 out]
          }
          frame "Compressor", "Digital Out" {
            w342 = FALSE ("Visible")
            # "Get direction and finish"
            n183 = property on="Motor" class="Clust (strict)"("Visible"=w342) -> ()  [unwired: 2 in, 2 out]
            n184 = property on="Test Slider" class="Slide (strict)"("Visible"=w342) -> ()  [unwired: 2 in, 2 out]
            n185 = property on="Test Ring" class="Ring (strict)"("Visible"=w342) -> ()  [unwired: 2 in, 2 out]
            n186 = property on="On/Off" class="Bool (strict)"("Visible"=TRUE, "Caption.Text"=w343) -> ()  [unwired: 2 in, 2 out]
            n187 = property on="Rev/Fwd" class="Clust (strict)"("Visible"=FALSE) -> ()  [unwired: 2 in, 2 out]
          }
          frame "Camera" {
            n188 = call <vilib>:"Get Last Path Segment.vi"("String in"=w350) -> ("String out"=w351:string)  [unwired: 10 in]
            n189 = property on="On/Off" class="Bool (strict)"("Visible"=FALSE) -> ()  [unwired: 2 in, 2 out]
            n190 = property on="Motor" class="Clust (strict)"("Visible"=FALSE) -> ()  [unwired: 2 in, 2 out]
            n191 = property on="Rev/Fwd" class="Clust (strict)"("Visible"=FALSE) -> ()  [unwired: 2 in, 2 out]
            n192 = case shown="\"White Balance  **\"" w351 {
              tunnel: w350 -> [w357 w366 w375 w384 w393 _ w399]
              tunnel: w349 -> [w355 w363 w372 w381 w390 _ _]
              frame "Size  **" {
                n193 = Index Array(array=w355) -> (element=w354:cluster{string[]})  [unwired: 1 in]
                n194 = call <vilib>:"NT Read String.vi"("Name"=w357) -> ("String"=w356:string)  [unwired: 9 in, 1 out]
                n195 = Unbundle(w354) -> (w352:string[])
                n196 = Match First String(2:w352, 3:w356) -> (0:w353:i32)  [unwired: 1 out]
                n197 = property on="Test Ring" class="Ring (strict)"("Value"=w353, "Strings []"=w352) -> ()  [unwired: 2 in, 2 out]
                n198 = property on="Test Ring" class="Ring (strict)"("Visible"=TRUE) -> ()  [unwired: 2 in, 2 out]
                n199 = property on="Test Slider" class="Slide (strict)"("Visible"=FALSE) -> ()  [unwired: 2 in, 2 out]
              }
              frame "White Balance  **" {
                n200 = Index Array(array=w363, index=1) -> (element=w364:cluster{string[]})
                n201 = call <vilib>:"NT Read String.vi"("Name"=w366) -> ("String"=w365:string)  [unwired: 9 in, 1 out]
                n202 = Unbundle(w364) -> (w361:string[])
                n203 = Match First String(2:w361, 3:w365) -> (0:w360:i32)  [unwired: 1 out]
                n204 = property on="Test Ring" class="Ring (strict)"("Value"=w360, "Strings []"=w361) -> ()  [unwired: 2 in, 2 out]
                n205 = property on="Test Ring" class="Ring (strict)"("Visible"=TRUE) -> ()  [unwired: 2 in, 2 out]
                n206 = property on="Test Slider" class="Slide (strict)"("Visible"=FALSE) -> ()  [unwired: 2 in, 2 out]
              }
              frame "Exposure  **" {
                n207 = Index Array(array=w372, index=2) -> (element=w373:cluster{string[]})
                n208 = call <vilib>:"NT Read String.vi"("Name"=w375) -> ("String"=w374:string)  [unwired: 9 in, 1 out]
                n209 = Unbundle(w373) -> (w369:string[])
                n210 = Match First String(2:w369, 3:w374) -> (0:w370:i32)  [unwired: 1 out]
                n211 = property on="Test Ring" class="Ring (strict)"("Value"=w370, "Strings []"=w369) -> ()  [unwired: 2 in, 2 out]
                n212 = property on="Test Ring" class="Ring (strict)"("Visible"=TRUE) -> ()  [unwired: 2 in, 2 out]
                n213 = property on="Test Slider" class="Slide (strict)"("Visible"=FALSE) -> ()  [unwired: 2 in, 2 out]
              }
              frame "Exposure Priority  **" {
                n214 = Index Array(array=w381, index=3) -> (element=w382:cluster{string[]})
                n215 = call <vilib>:"NT Read String.vi"("Name"=w384) -> ("String"=w383:string)  [unwired: 9 in, 1 out]
                n216 = Unbundle(w382) -> (w378:string[])
                n217 = Match First String(2:w378, 3:w383) -> (0:w379:i32)  [unwired: 1 out]
                n218 = property on="Test Ring" class="Ring (strict)"("Value"=w379, "Strings []"=w378) -> ()  [unwired: 2 in, 2 out]
                n219 = property on="Test Ring" class="Ring (strict)"("Visible"=TRUE) -> ()  [unwired: 2 in, 2 out]
                n220 = property on="Test Slider" class="Slide (strict)"("Visible"=FALSE) -> ()  [unwired: 2 in, 2 out]
              }
              frame "Color Enable  **" {
                n221 = Index Array(array=w390, index=4) -> (element=w391:cluster{string[]})
                n222 = call <vilib>:"NT Read String.vi"("Name"=w393) -> ("String"=w392:string)  [unwired: 9 in, 1 out]
                n223 = Unbundle(w391) -> (w387:string[])
                n224 = Match First String(2:w387, 3:w392) -> (0:w388:i32)  [unwired: 1 out]
                n225 = property on="Test Ring" class="Ring (strict)"("Value"=w388, "Strings []"=w387) -> ()  [unwired: 2 in, 2 out]
                n226 = property on="Test Ring" class="Ring (strict)"("Visible"=TRUE) -> ()  [unwired: 2 in, 2 out]
                n227 = property on="Test Slider" class="Slide (strict)"("Visible"=FALSE) -> ()  [unwired: 2 in, 2 out]
              }
              frame Default {
                n228 = property on="Test Ring" class="Ring (strict)"("Visible"=FALSE) -> ()  [unwired: 2 in, 2 out]
                n229 = property on="Test Slider" class="Slide (strict)"("Visible"=FALSE) -> ()  [unwired: 2 in, 2 out]
              }
              frame "Brightness  **", "Color Level  **", "Compression  **", "FPS  **", "Sharpness  **" {
                n230 = call <vilib>:"NT Read Number.vi"("Name"=w399) -> ("Numeric"=w398:dbl)  [unwired: 9 in, 1 out]
                n231 = local write "Test Slider"(w398) -> ()
                n232 = property on="Test Slider" class="Slide (strict)"("Visible"=TRUE, "Scale.Maximum"=100.0 ("Scale.Range:Maximum")) -> ()  [unwired: 2 in, 2 out]
                n233 = property on="Test Ring" class="Ring (strict)"("Visible"=FALSE) -> ()  [unwired: 2 in, 2 out]
              }
            }
          }
        }
        n234 = property on="Progress" class="Clust (strict)"("Visible"=FALSE) -> ()  [unwired: 2 in, 2 out]
      }
      event "Test Name": Mouse Enter {
        # "Populate the ring with the list of tests"
        n235 = event-data() -> ()  [unwired: 1 in, 1 out]
        n236 = call <vilib>:"NT Read String Array.vi"("Name"="TestMode/TestList") -> ("String Array"=w407:string[])  [unwired: 9 in, 1 out]
        n237 = Build Array (concatenate)("Select the test to run...", w407) -> (w406:string[])
        n238 = property on="Test Name" class="Ring (strict)"("Strings []"=w406) -> ()  [unwired: 2 in, 2 out]
      }
      event "Test Name": Value Change {
        w409 = FALSE ("Visible")
        # "Tell the robot the test name to run"
        n239 = event-data() -> ("NewVal"=w413:u16)  [unwired: 1 in]
        n240 = property on="Test Name" class="Ring (strict)"() -> ("Strings []"=w414:string[])  [unwired: 2 in, 2 out]
        n241 = local write "Progress"(T7 {"Test Progress"=0, "Test Progress Text"=""} ("Progress")) -> ()
        n242 = Index Array(array=w414, index=w413) -> (element=w412:string)
        n243 = call <vilib>:"NT Write String.vi"("String"=w412, "Name"="TestMode/TestName") -> ()  [unwired: 9 in, 1 out]
        n244 = property on="Progress" class="Clust (strict)"("Visible"=TRUE) -> ()  [unwired: 2 in, 2 out]
        n245 = property on="Motor" class="Clust (strict)"("Visible"=w409) -> ()  [unwired: 2 in, 2 out]
        n246 = property on="Test Slider" class="Slide (strict)"("Visible"=w409) -> ()  [unwired: 2 in, 2 out]
        n247 = property on="On/Off" class="Bool (strict)"("Visible"=w409) -> ()  [unwired: 2 in, 2 out]
        n248 = property on="Rev/Fwd" class="Clust (strict)"("Visible"=w409) -> ()  [unwired: 2 in, 2 out]
        n249 = property on="Test Ring" class="Ring (strict)"("Visible"=w409) -> ()  [unwired: 2 in, 2 out]
      }
      event "Select Auto": Mouse Enter {
        # "Populate the combo box with the list of autonomous options"
        n250 = event-data() -> ()  [unwired: 1 in, 1 out]
        n251 = call <vilib>:"NT Read String Array.vi"("Name"="Auto List") -> ("String Array"=w416:string[])  [unwired: 9 in, 1 out]
        n252 = property on="Select Auto" class="CmbBox"("Strings[]"=w416) -> ()  [unwired: 2 in, 2 out]
      }
      event "Select Auto": Value Change {
        # "User modified the Auto Selection. Write to NT variable so robot knows."
        n253 = event-data() -> ("NewVal"=w419:string)  [unwired: 1 in]
        n254 = call <vilib>:"NT Write String.vi"("String"=w419, "Name"="Auto Selector") -> ()  [unwired: 9 in, 1 out]
      }
      event "Command Selection": Value Change {
        # "Get the params and show in table"
        n255 = event-data() -> ("NewVal"=w425:i32)  [unwired: 1 in]
        n256 = property on="Command Selection" class="MCListbox (strict)"() -> ("ItemNames"=w423:string[][])  [unwired: 2 in, 2 out]
        n257 = call <vilib>:"WPI_DashboardUpdate Command Params.vi"("NewVal"=w425, "Commands"=w423, "Param Tbl"=w424) -> ()  [unwired: 8 in, 1 out]
      }
      event "Execute Command": Value Change {
        # "Started one, Unique ID holds\nresponse"
        n258 = event-data() -> ()  [unwired: 1 in, 1 out]
        n259 = property on="Command Selection" class="MCListbox (strict)"() -> ("ItemNames"=w436:string[][])  [unwired: 2 in, 2 out]
        n260 = Index Array(array=w436, index (row)="Command Selection", index (col)=0) -> (element=w434:string)
        n261 = call <vilib>:"Invoke Commands.vi"("Command Params"="Command Params", "Function Name"=w434) -> ("Params"=w430:u8, "Started"=w429:bool)  [unwired: 7 in, 1 out]
        n262 = Array Subset(array="Command Params", length (row)=w430) -> (w431:string[][])  [unwired: 3 in]
        n263 = Select(t="Executing" ("Cmd Status"), s=w429, f="" ("Cmd Status")) -> (s? t:f=→"Cmd Status":string)
      }
      event "Command Selection": Double Click {
        n264 = event-data() -> ("Row"=w444:i32)  [unwired: 1 in]
        n265 = local read "Command Params"() -> (w443:string[][])
        n266 = property on="Command Selection" class="MCListbox (strict)"() -> ("ItemNames"=w447:string[][])  [unwired: 2 in, 2 out]
        n267 = Index Array(array=w447, index (row)=w444, index (col)=0) -> (element=w445:string)
        n268 = call <vilib>:"Invoke Commands.vi"("Command Params"=w443, "Function Name"=w445) -> ("Params"=w442:u8, "Started"=w437:bool)  [unwired: 7 in, 1 out]
        n269 = Array Subset(array=w443, length (row)=w442) -> (w441:string[][])  [unwired: 3 in]
        n270 = Select(t="Executing" ("Cmd Status"), s=w437, f="" ("Cmd Status")) -> (s? t:f=w438:string)
        n271 = local write "Cmd Status"(w438) -> ()
      }
      event "CheckList": Double Click {
        # "Shift clears all"
        # "Update symbols on the listbox"
        n272 = event-data() -> ("PlatMods.Shift"=w449:bool, "Row"=w451:i32)  [unwired: 1 in]
        n273 = case shown="True" w449 {
          tunnel: w451 -> [w455 _]
          tunnel: 1 -> [w454 _]
          frame False {
            n274 = property on="CheckList" class="LstBox (strict)"() -> ("Item Symbols"=w453:i32[])  [unwired: 2 in, 2 out]
            n275 = Replace Array Subset(array=w453, new element=w454, index=w455) -> (w452:i32[])
            n276 = property on="CheckList" class="LstBox (strict)"("Item Symbols"=w452) -> ()  [unwired: 2 in, 2 out]
          }
          frame True {
            w456 = 0 ("Top Row")
            n277 = property on="CheckList" class="LstBox (strict)"() -> ("Number of Rows"=w458:u32)  [unwired: 2 in, 2 out]
            n278 = Initialize Array(0, w458) -> (w457:i32[])
            n279 = property on="CheckList" class="LstBox (strict)"("Top Row"=w456, "Value"=w456, "Item Symbols"=w457) -> ()  [unwired: 2 in, 2 out]
          }
        }
      }
      event "CheckList": Key Down {
        # "Update symbols on the listbox\nLeft and right keys check and uncheck"
        n280 = event-data() -> ("VKey"=w462:T26)  [unwired: 1 in]
        n281 = case shown="\"Left\", \"Right\"" w462 {
          selector: w462 -> [w467 _]
          tunnel: eventvkey."Left" ("VKey") -> [w465 _]
          frame "Left", "Right" {
            n282 = Equal?(x=w465, y=w467) -> (x = y?=w466:bool)
            n283 = Select(t=0, s=w466, f=1) -> (s? t:f=w468:i32)
            n284 = property on="CheckList" class="LstBox (strict)"() -> ("Item Symbols"=w471:i32[])  [unwired: 2 in, 2 out]
            n285 = Replace Array Subset(array=w471, new element=w468, index="CheckList") -> (w470:i32[])
            n286 = property on="CheckList" class="LstBox (strict)"("Item Symbols"=w470) -> ()  [unwired: 2 in, 2 out]
          }
          frame Default {
          }
        }
      }
      event "Motor.Enable": Value Change {
        # "When the test mode otor enable helper is set, update that\ntree row item's value"
        n287 = event-data() -> ("NewVal"=w477:bool)  [unwired: 1 in]
        n288 = Unbundle("Motor") -> ("Value"=w476:dbl)  [unwired: 1 out]
        n289 = Select(t=w476, s=w477, f=0.0) -> (s? t:f=w474:dbl)
        n290 = call <vilib>:"NT Write Number.vi"("Numeric"=w474, "Name"=w473) -> ()  [unwired: 9 in, 1 out]
      }
      event "Test Slider": Value Change {
        # "When the test mode slider helper is set, update that\ntree row item's value"
        n291 = event-data() -> ("NewVal"=w480:dbl)  [unwired: 1 in]
        n292 = call <vilib>:"NT Write Number.vi"("Numeric"=w480, "Name"=w481) -> ()  [unwired: 9 in, 1 out]
      }
      event "On/Off": Value Change {
        # "When the test mode on/off helper value is set, update that\ntree row item's value"
        n293 = event-data() -> ("NewVal"=w485:bool)  [unwired: 1 in]
        n294 = Boolean To (0,1)(Boolean=w485) -> (0, 1=w484:i16)
        n295 = call <vilib>:"NT Write Number.vi"("Numeric"=w484, "Name"=w483) -> ()  [unwired: 9 in, 1 out]
      }
      event "Rev/Fwd": Value Change {
        # "When the test mode helper value for relays is set, update that\ntree row item's value"
        n296 = event-data() -> ("NewVal.Forward"=w493:bool, "NewVal.Reverse"=w492:bool)  [unwired: 1 in]
        n297 = Boolean To (0,1)(Boolean=w493) -> (0, 1=w489:i16)
        n298 = Boolean To (0,1)(Boolean=w492) -> (0, 1=w491:i16)
        n299 = Negate(x=w491) -> (-x=w490:i16)
        n300 = Add(x=w489, y=w490) -> (x+y=w488:i16)
        n301 = call <vilib>:"NT Write Number.vi"("Numeric"=w488, "Name"=w487) -> ()  [unwired: 9 in, 1 out]
      }
      event "Test Ring": Value Change {
        # "When a test mode helper value is selected from the ring,\nset the tree item's variable to the string value"
        n302 = event-data() -> ("NewVal"=w497:u16)  [unwired: 1 in]
        n303 = property on="Test Ring" class="Ring (strict)"() -> ("Strings []"=w498:string[])  [unwired: 2 in, 2 out]
        n304 = Index Array(array=w498, index=w497) -> (element=w496:string)
        n305 = call <vilib>:"NT Write String.vi"("String"=w496, "Name"=w495) -> ()  [unwired: 9 in, 1 out]
      }
      event "Rec Mode": Value Change {
        # "Update globals for recording mode and path to read log from.\nClear when logging and let NetworkTables set path for vision to\nuse."
        n306 = event-data() -> ("NewVal"=w509:enum32{"Stop", "Record", "Playback"})  [unwired: 1 in]
        n307 = global write "WPI_DashboardLogging Global.vi" "Logging Filename"(path "") -> ()
        n308 = global write "WPI_DashboardLogging Global.vi" "Recording"(w509) -> ()
        n309 = case shown="\"Playback\"" w509 {
          tunnel: w508 -> [_ w511 w520]
          tunnel: [_ _ w519] -> w506
          tunnel: [_ _ w518] -> _
          tunnel: w504 -> [_ _ w516]
          tunnel: cluster{i32, i32} {-250, 170} -> [_ _ w515]
          tunnel: [_ _ T27 {"Image Size"=TRUE, "Image Type"=TRUE, "Pixel Value"=TRUE, "ROI Information"=TRUE, "Zoom Factor"=FALSE} ("Image Information Shown:All Elements")] -> w499
          tunnel: [_ _ TRUE ("Zoom Factor")] -> w500
          tunnel: w502 -> [_ _ w512]
          frame Default {
          }
          frame "Stop", "Record" {
            # "Place Window too"
            n310 = invoke class="VI" method="FP.Close"(reference=w511) -> (reference out=w510:refnum<vi>)  [unwired: 2 in, 2 out]
            n311 = invoke class="VI" method="Abort VI"(reference=w510) -> ()  [unwired: 2 in, 3 out]
          }
          frame "Playback" {
            n312 = call "Open Playback Panel.vi"("Offset"=w515, "DB VI Ref"=w516, "Playback in"=w520) -> ("Playback out"=w517:refnum<vi>)  [unwired: 8 in]
            n313 = register-events(w517, w512) -> (reference out=w519:refnum<event-registration>, error out=w518:errorcluster)  [unwired: 2 in]
          }
        }
        n314 = property on="Camera Image Right" class="ImageControl"("Image Information Shown"=w499, "Image Information Visible"=w500) -> ()  [unwired: 2 in, 2 out]
        n315 = property on="Camera Image" class="ImageControl"("Image Information Shown"=w499, "Image Information Visible"=w500) -> ()  [unwired: 2 in, 2 out]
        n316 = call <vilib>:"WPI_DashboardNT Log FieldName Cache.vi"("Operation"=enum16{"Lookup/Add", "Index", "Clear"}."Clear") -> ()  [unwired: 8 in, 3 out]
      }
      event Panel Close {
        w522 = enum32{"Stop", "Record", "Playback"}."Stop" ("Rec Mode")
        # "Playback window has been closed, abort"
        n317 = event-data() -> ()  [unwired: 1 in, 4 out]
        n318 = local write "Rec Mode"(w522) -> ()
        n319 = global write "WPI_DashboardLogging Global.vi" "Recording"(w522) -> ()
      }
      event Panel Close {
        # "Abort playback window and ourself"
        n320 = event-data() -> ()  [unwired: 1 in, 4 out]
        n321 = invoke class="VI" method="FP.Close"(reference=w526) -> (reference out=w525:refnum<vi>)  [unwired: 2 in, 2 out]
        n322 = invoke class="VI" method="Abort VI"(reference=w525) -> (error out=w524:errorcluster)  [unwired: 2 in, 2 out]
        n323 = invoke class="VI" method="Abort VI"(error in=w524) -> ()  [unwired: 2 in, 3 out]
      }
      event User Event {
        n324 = event-data() -> ("IDs"=w533:cluster{"RPC field ID":u16, "Unique ID":u16}, "String"=w532:string)  [unwired: 1 in]
        n325 = Bundle("IDs"=w533, "String"=w532) -> (w531:T10)  [unwired: 1 in]
        n326 = call <vilib>:"Retrieve RPC Response.vi"("RPC Response"=w531) -> ("Output"=w529:string[][])  [unwired: 10 in]
        n327 = Build Array (concatenate)(w527, w529) -> (w528:string[][])
        n328 = local write "Command Params"(w528) -> ()
        n329 = local write "Cmd Status"("" ("Cmd Status")) -> ()
      }
      event "Tree": Double Click {
        n330 = event-data() -> ("PlatMods"=w539:T30, "Tag"=w536:string)  [unwired: 1 in]
        n331 = Unbundle(w539) -> ("Shift"=w538:bool)  [unwired: 4 out]
        n332 = String Subset(string=w536, length (rest)=1 ("length (rest)")) -> (substring=w535:string)  [unwired: 1 in]
        n333 = Not(x=w538) -> (.not. x?=w537:bool)
        n334 = case shown="\"/\"" w535 {
          tunnel: w536 -> [_ w542]
          tunnel: w537 -> [_ w541]
          frame Default {
          }
          frame "/" {
            n335 = call <vilib>:"NT Update Persistence.vi"("Persistence"=w541, "Name"=w542) -> ()  [unwired: 9 in, 1 out]
          }
        }
      }
    }
  }
  n336 = local write "Dashboard Tab"(T2."Drive" ("Dashboard Tab")) -> ()
  n337 = property on="On/Off" class="Bool (strict)"("Visible"=w37) -> ()  [unwired: 2 in, 2 out]
  n338 = property on="Motor" class="Clust (strict)"("Visible"=w37) -> ()  [unwired: 2 in, 2 out]
  n339 = property on="Progress" class="Clust (strict)"("Visible"=w37) -> ()  [unwired: 2 in, 2 out]
  n340 = property on="Test Ring" class="Ring (strict)"("Visible"=w37) -> ()  [unwired: 2 in, 2 out]
  n341 = property on="Rev/Fwd" class="Clust (strict)"("Visible"=w37) -> ()  [unwired: 2 in, 2 out]
  n342 = while {
    tunnel: u16 1741 ("timeout ms (25000)") -> [w544]
    stop <- FALSE stop-if-true
    n343 = TCP Create Listener(10:w544) -> (0:w543:errorcluster, 3:w545:refnum<k5>)  [unwired: 4 in, 1 out]
    n344 = case shown="No Error" w543 {
      selector: w543 -> [w547 _]
      tunnel: w545 -> [w548 _]
      frame No Error {
        n345 = while {
          tunnel: w548 -> [w551]
          tunnel: w547 -> [w550]
          stop <- FALSE stop-if-true
          n346 = TCP Wait On Listener(8:w550, 11:w551) -> (0:w552:errorcluster, 4:w553:refnum<k5>)  [unwired: 2 in, 3 out]
          n347 = local write "TCP"(w553) -> ()
          n348 = case shown="No Error" w552 {
            frame No Error {
            }
            frame Error {
              n349 = Wait (ms)(milliseconds to wait=u32 1000) -> ()  [unwired: 1 out]
            }
          }
        }
      }
      frame Error {
        n350 = Wait (ms)(milliseconds to wait=u32 1000) -> ()  [unwired: 1 out]
      }
    }
  }
  n351 = local write "Command Selection"(u16 0 ("milliseconds to wait")) -> ()
  n352 = local write "Command Params"(string[][] [] ("Command Params")) -> ()
  n353 = global write "WPI_DashboardLogging Global.vi" "Recording"(w60) -> ()
  n354 = local write "Rec Mode"(w60) -> ()
  n355 = call <vilib>:"NT Write String.vi"("String"="Select Auto", "Name"="Auto Selector") -> ()  [unwired: 9 in, 1 out]
